vi "DHT_Final.vi"() -> ()   [LabVIEW 2020]
panel:
  in  "VISA resource name":refnum<visa-resource-name>
  in  "Table Control":string[][](table)
  out "Humidity":dbl(graph)
  out "Temp":dbl(graph)
  out "Humdity":dbl(knob) scale=0.0..100.0
  out "Temp":dbl(slide) scale=0.0..50.0
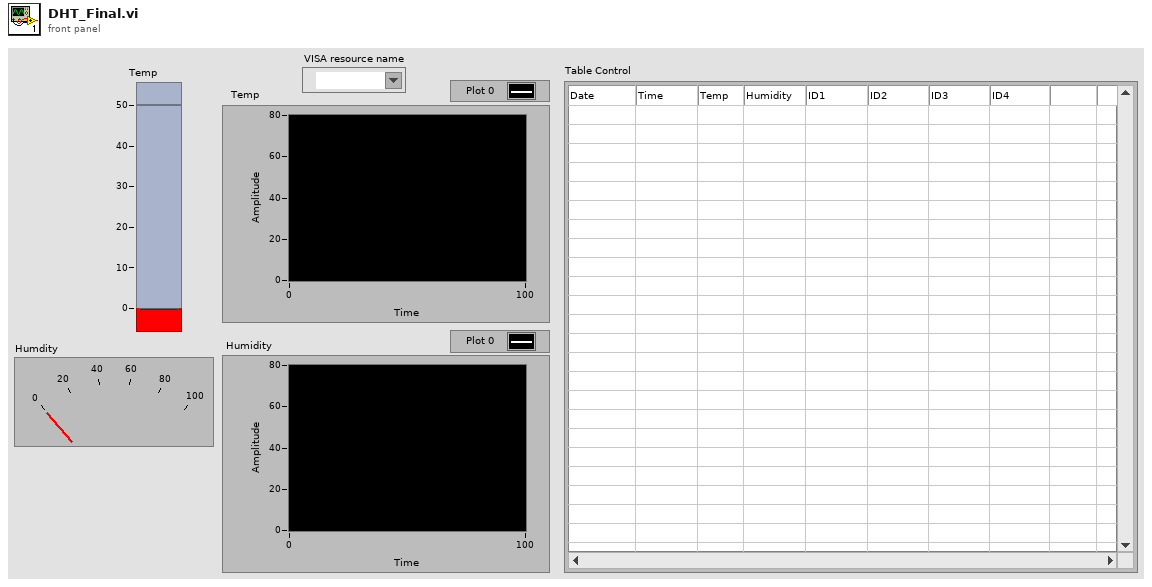
[diagram p1: front panel]
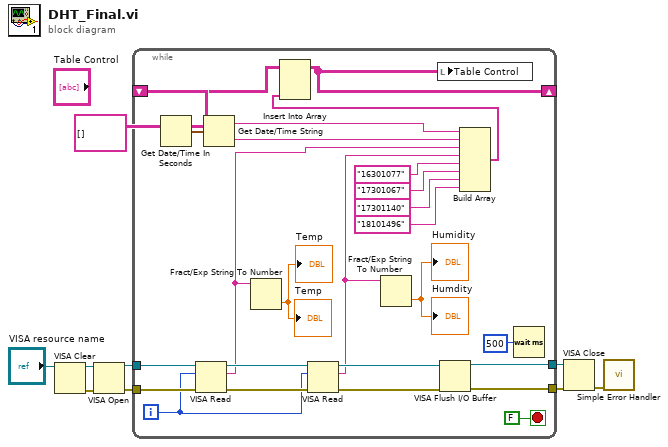
[diagram p0: block diagram]
diagram:
  n1 = VISA Clear(VISA resource name="VISA resource name") -> (VISA resource name out=w8:refnum<visa-resource-name>, error out=w9:errorcluster)  [unwired: 1 in]
  n2 = VISA Open(error in (no error)=w9, VISA resource name=w8) -> (VISA resource name=w6:refnum<visa-resource-name>, error out=w5:errorcluster)  [unwired: 3 in]
  n3 = while {
    tunnel: w6 -> [w30]
    tunnel: w5 -> [w34]
    tunnel: [w31] -> w4
    tunnel: [w27] -> w3
    shift-right: [w11] -> _
    shift-left: string[][] [] -> [w21]
    i -> [w22]
    stop <- FALSE stop-if-true
    n4 = Get Date/Time In Seconds() -> (seconds since 1Jan1904=w25:timestamp)
    n5 = VISA Read(VISA resource name=w30, byte count=w22, error in (no error)=w34) -> (VISA resource name out=w29:refnum<visa-resource-name>, read buffer=w13:string, error out=w33:errorcluster)  [unwired: 1 out]
    n6 = Get Date/Time String(seconds (now)=w25) -> (date string=w20:string, time string=w19:string)  [unwired: 2 in]
    n7 = Fract/Exp String To Number(string=w13) -> (number=→"Temp" →"Temp":dbl)  [unwired: 3 in, 1 out]
    n8 = VISA Read(VISA resource name=w29, byte count=w22, error in (no error)=w33) -> (VISA resource name out=w28:refnum<visa-resource-name>, read buffer=w14:string, error out=w32:errorcluster)  [unwired: 1 out]
    n9 = Fract/Exp String To Number(string=w14) -> (number=→"Humdity" →"Humidity":dbl)  [unwired: 3 in, 1 out]
    n10 = VISA Flush I/O Buffer(VISA resource name=w28, error in (no error)=w32) -> (VISA resource name out=w27:refnum<visa-resource-name>, error out=w31:errorcluster)  [unwired: 1 in]
    n11 = Build Array(w20, w19, w13, w14, "16301077" ("element"), "17301067" ("element"), "17301140", "18101496" ("element")) -> (w15:string[])
    n12 = Insert Into Array(array=w21, new element=w15) -> (w11:string[][])  [unwired: 2 in]
    n13 = local write "Table Control"(w11) -> ()
    n14 = Wait (ms)(milliseconds to wait=u32 500) -> ()  [unwired: 1 out]
  }
  n15 = VISA Close(VISA resource name=w3, error in (no error)=w4) -> (error out=w7:errorcluster)
  n16 = call <vilib>:"Simple Error Handler.vi"("error in (no error)"=w7) -> ()  [unwired: 4 in, 5 out]
